vi "Create File with Incrementing Suffix.vi"(6 "disable buffering (F)":bool, 7 "format string (\" (%d)\")":string=" (%d)", 8 "error in (no error)":errorcluster, 11 "file path":path) -> (0 "error out":errorcluster, 2 "actual path":path)   [LabVIEW 2015]
doc: "Creates a file and appends an incrementing number suffix to the filename if the file already exists at a specified path. If the file does not exist, this VI creates the file without appending an incrementing number suffix to the filename."
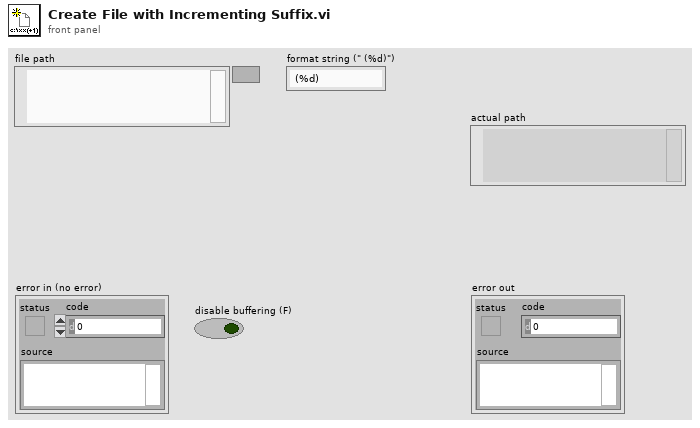
[diagram p1: front panel]
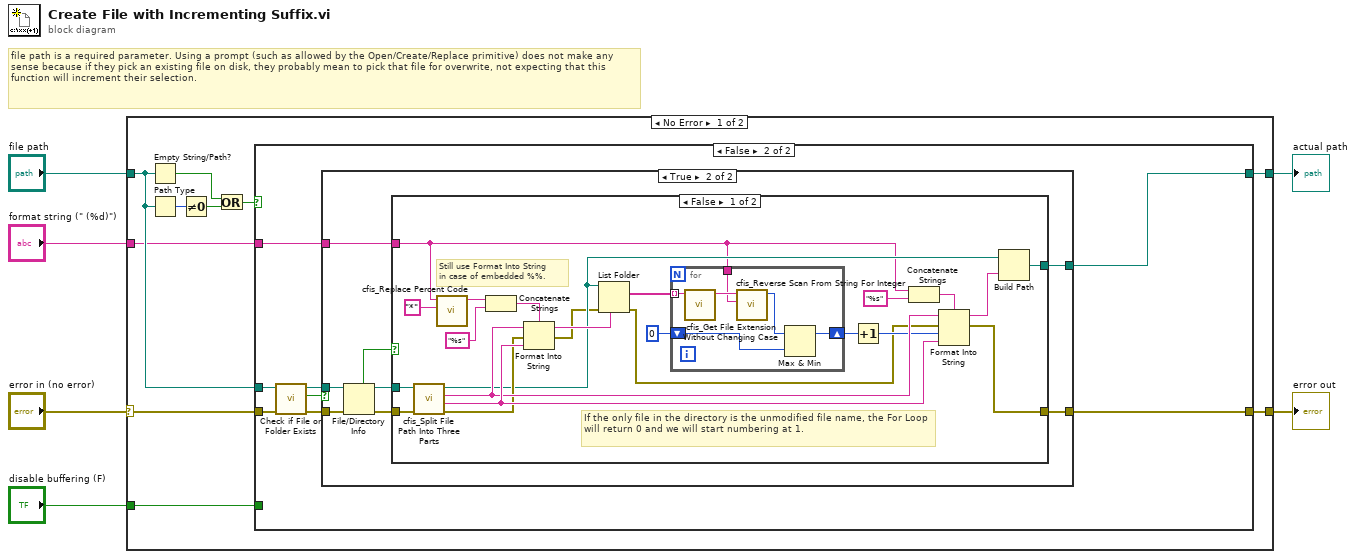
[diagram p0: block diagram]
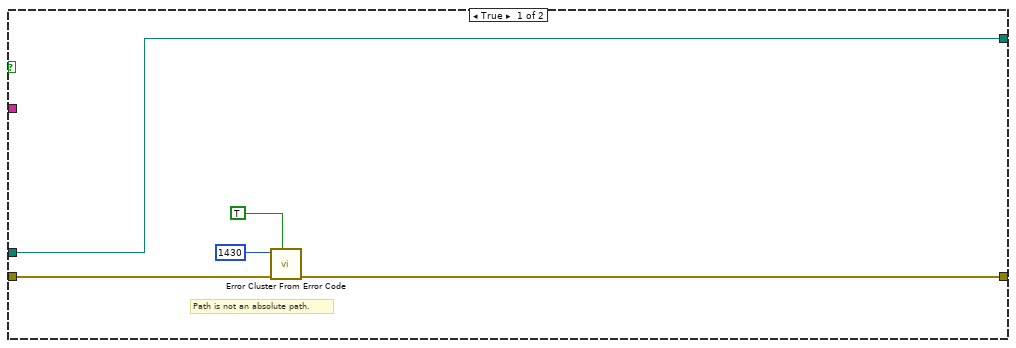
[diagram p2: hidden frame]
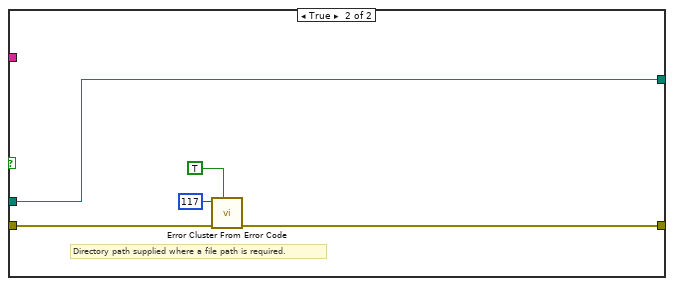
[diagram p4: hidden frame]
diagram:
  # "file path is a required parameter. Using a prompt (such as allowed by the Open/Create/Replace primitive) does not make any sense because if they pick an existing file on disk, they probably mean to pick that file for overwrite, not expecting that this function will increment their selection."
  n1 = case shown="No Error" "error in (no error)" {
    selector: "error in (no error)" -> [w14 w74]
    tunnel: "file path" -> [w9 w73]
    tunnel: "disable buffering (F)" -> [w16 _]
    tunnel: [w15 w74] -> w4
    tunnel: [w8 w73] -> w2
    tunnel: "format string (\" (%d)\")" -> [w7 _]
    frame No Error {
      n2 = Empty String/Path?(string/path=w9) -> (empty?=w11:bool)
      n3 = Path Type(1:w9) -> (0:w13:i16)
      n4 = Not Equal To 0?(x=w13) -> (x != 0?=w12:bool)
      n5 = Or(x=w11, y=w12) -> (x .or. y?=w10:bool)
      n6 = case shown="False" w10 {
        tunnel: w16 -> [_ _]
        tunnel: [w21 w22] -> w15
        tunnel: w14 -> [w19 w29]
        tunnel: w9 -> [w17 w28]
        tunnel: [w17 w23] -> w8
        tunnel: w7 -> [_ w24]
        frame True {
          # "Path is not an absolute path."
          n7 = call <vilib>:"Error Cluster From Error Code.vi"("show call chain? (False)"=TRUE, "error in (no error)"=w19, "error code (0)"=1430) -> ("error out"=w21:errorcluster)  [unwired: 6 in]
        }
        frame False {
          n8 = call <vilib>:"Check if File or Folder Exists.vi"("error in (no error)"=w29, "path"=w28) -> ("error out"=w25:errorcluster, "file or folder exists?"=w27:bool, "dup path"=w26:path)  [unwired: 7 in]
          n9 = case shown="True" w27 {
            tunnel: w26 -> [w31 w39]
            tunnel: [w31 w33] -> w23
            tunnel: w25 -> [w30 w38]
            tunnel: [w30 w35] -> w22
            tunnel: w24 -> [_ w32]
            frame False {
            }
            frame True {
              n10 = File/Directory Info(path=w39, error in=w38) -> (path out=w34:path, directory=w37:bool, error out=w36:errorcluster)  [unwired: 4 out]
              n11 = case shown="False" w37 {
                tunnel: w36 -> [w52 w72]
                tunnel: [w42 w69] -> w35
                tunnel: w34 -> [w61 w68]
                tunnel: [w43 w68] -> w33
                tunnel: w32 -> [w40 _]
                frame False {
                  # "If the only file in the directory is the unmodified file name, the For Loop will return 0 and we will start numbering at 1."
                  # "Still use Format Into String\nin case of embedded %%."
                  n12 = call <vilib>:"cfis_Split File Path Into Three Parts.vi"("file path"=w61) -> ("File extension"=w54:string, "File name without extension"=w53:string, "Directory"=w50:path)  [unwired: 8 in]
                  n13 = call <vilib>:"cfis_Replace Percent Code.vi"("replace text"="*", "format string in"=w40) -> ("format string out"=w57:string)  [unwired: 9 in]
                  n14 = Concatenate Strings(w57, "%s" ("format string")) -> (w56:string)
                  n15 = Format Into String(format string=w56, initial string=w53, error in=w52, w54) -> (resulting string=w51:string, error out=w49:errorcluster)
                  n16 = List Folder(path=w50, pattern=w51, error in=w49) -> (filenames=w48:string[], error out=w41:errorcluster)  [unwired: 1 in, 2 out]
                  n17 = for {
                    tunnel: w48 -> [w67] mode=indexing
                    shift-right: [w63] -> w46
                    shift-left: 0 -> [w64]
                    tunnel: w40 -> [w62]
                    n18 = call <vilib>:"cfis_Get File Extension Without Changing Case.vi"("file name"=w67) -> ("file name without extension"=w66:string)  [unwired: 9 in, 1 out]
                    n19 = call <vilib>:"cfis_Reverse Scan From String For Integer.vi"("format string"=w62, "input string"=w66) -> ("Extracted integer"=w65:i32)  [unwired: 9 in]
                    n20 = Max & Min(x=w65, y=w64) -> (max(x,y)=w63:i32)  [unwired: 1 out]
                  }
                  n21 = Increment(x=w46) -> (x+1=w44:i32)
                  n22 = Concatenate Strings(w40, "%s" ("format string")) -> (w59:string)
                  n23 = Format Into String(format string=w59, initial string=w53, error in=w41, w44, w54) -> (resulting string=w45:string, error out=w42:errorcluster)
                  n24 = Build Path(base path=w50, name or relative path=w45) -> (appended path=w43:path)
                }
                frame True {
                  # "Directory path supplied where a file path is required."
                  n25 = call <vilib>:"Error Cluster From Error Code.vi"("show call chain? (False)"=TRUE, "error in (no error)"=w72, "error code (0)"=117) -> ("error out"=w69:errorcluster)  [unwired: 6 in]
                }
              }
            }
          }
        }
      }
    }
    frame Error {
    }
  }
  "error out" <- w4
  "actual path" <- w2
